vi "CSC_InitCuffParam.vi"(6 "Shank":T2={"Center of Mass in LCS"={"Coord4"=[0.0, 0.0, 0.0, 1.0], "ID"=0}, "Mass"=0.0, "Cable Attachment Points in LCS"=[]} {"Mass" format="%#_13g"}, 8 "error in (no error)":errorcluster, 9 "Thigh":T2={"Center of Mass in LCS"={"Coord4"=[0.0, 0.0, 0.0, 1.0], "ID"=0}, "Mass"=0.0, "Cable Attachment Points in LCS"=[]} {"Mass" format="%#_13g"}, 10 "Pelvis":T2={"Center of Mass in LCS"={"Coord4"=[0.0, 0.0, 0.0, 1.0], "ID"=0}, "Mass"=0.0, "Cable Attachment Points in LCS"=[]} {"Mass" format="%#_13g"}, 11 "C-Alex in":refnum<class "CableSerialChain.lvclass">) -> (0 "error out":errorcluster, 3 "C-Alex out":refnum<class "CableSerialChain.lvclass">)   [LabVIEW 2014]
uses:
  Body/PointOnBody.ctl
  Body/Bodies.lvclass
  TypeDef/Cuff.ctl
  CableSerialChain.lvclass
panel:
  in  "Gravitaty(9.8)":dbl=9.806
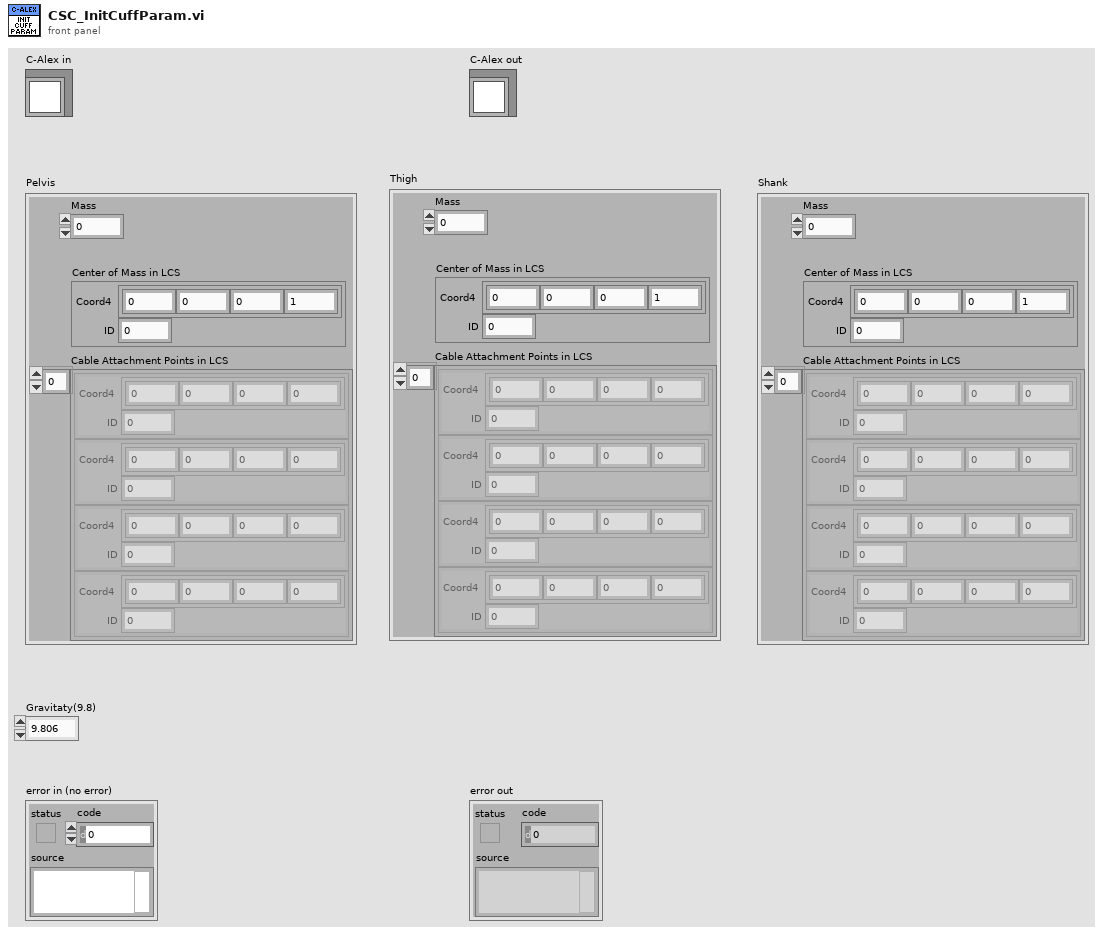
[diagram p1: front panel]
types:
  T1 = typedef "Bodies.lvclass/PointOnBody.ctl" = cluster{"Coord4":dbl[], "ID":i32}
  T2 = cluster{"Center of Mass in LCS":T1, "Mass":dbl, "Cable Attachment Points in LCS":T1[]}
  T3 = typedef "CableSerialChain.lvclass/Cuff.ctl" = cluster{"BodyID":i32, "OriginInLegCoSys":T1, "CoMInCuffCoSys":T1, "CoMInLegCoSys":T1, "Weight(N)":dbl, "CableAttPtsInCuffCoSys":T1[]}
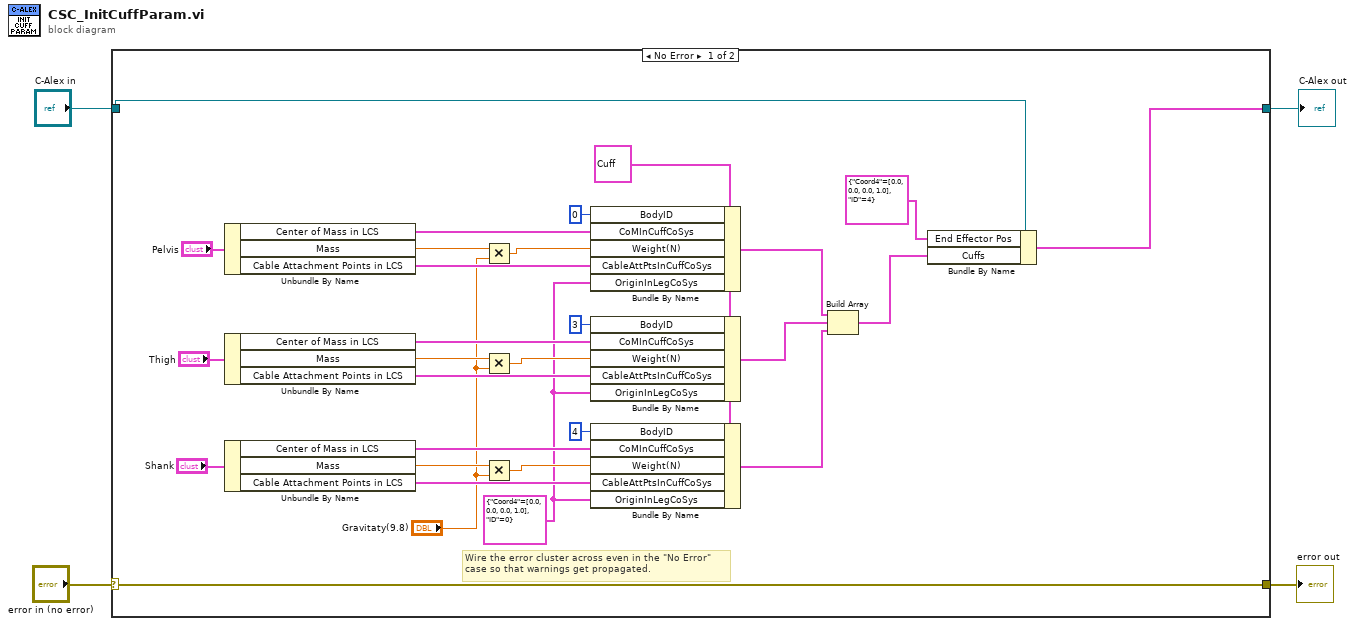
[diagram p0: block diagram]
diagram:
  n1 = case shown="No Error" "error in (no error)" {
    selector: "error in (no error)" -> [w33 w35]
    tunnel: [w33 w35] -> w3
    tunnel: [w31 w34] -> w1
    tunnel: "C-Alex in" -> [w32 w34]
    frame No Error {
      w5 = T1 {"Coord4"=[0.0, 0.0, 0.0, 1.0], "ID"=0} ("OriginInLegCoSys")
      w20 = T3 {"BodyID"=0, "OriginInLegCoSys"={"Coord4"=[], "ID"=0}, "CoMInCuffCoSys"={"Coord4"=[], "ID"=0}, "CoMInLegCoSys"={"Coord4"=[], "ID"=0}, "Weight(N)"=0.0, "CableAttPtsInCuffCoSys"=[]} ("CuffConstant")
      # "Wire the error cluster across even in the \"No Error\"\ncase so that warnings get propagated."
      n2 = Unbundle By Name("Pelvis") -> ("Center of Mass in LCS"=w28:T1, "Mass"=w10:dbl, "Cable Attachment Points in LCS"=w29:T1[])
      n3 = Unbundle By Name("Thigh") -> ("Center of Mass in LCS"=w27:T1, "Mass"=w12:dbl, "Cable Attachment Points in LCS"=w26:T1[])
      n4 = Unbundle By Name("Shank") -> ("Center of Mass in LCS"=w21:T1, "Mass"=w15:dbl, "Cable Attachment Points in LCS"=w22:T1[])
      n5 = Multiply(x=w10, y="Gravitaty(9.8)") -> (x*y=w11:dbl)
      n6 = Multiply(x=w12, y="Gravitaty(9.8)") -> (x*y=w13:dbl)
      n7 = Multiply(x=w15, y="Gravitaty(9.8)") -> (x*y=w14:dbl)
      n8 = Bundle By Name(cluster=w20, "BodyID"=0, "CoMInCuffCoSys"=w28, "Weight(N)"=w11, "CableAttPtsInCuffCoSys"=w29, "OriginInLegCoSys"=w5) -> (w16:T3)
      n9 = Bundle By Name(cluster=w20, "BodyID"=3, "CoMInCuffCoSys"=w27, "Weight(N)"=w13, "CableAttPtsInCuffCoSys"=w26, "OriginInLegCoSys"=w5) -> (w17:T3)
      n10 = Bundle By Name(cluster=w20, "BodyID"=4, "CoMInCuffCoSys"=w21, "Weight(N)"=w14, "CableAttPtsInCuffCoSys"=w22, "OriginInLegCoSys"=w5) -> (w18:T3)
      n11 = Build Array(w16, w17, w18) -> (w8:T3[])
      n12 = Bundle By Name(cluster=w32, "End Effector Pos"=T1 {"Coord4"=[0.0, 0.0, 0.0, 1.0], "ID"=4}, "Cuffs"=w8) -> (w31:cluster{})
    }
    frame Error {
    }
  }
  "error out" <- w3
  "C-Alex out" <- w1
